vi "MongoDB.Database.CreateCollection.vi"(8 "error in (no error)":errorcluster, 11 "MongoDB.Database in":refnum<class "MongoDB.Database.lvclass">) -> (0 "error out":errorcluster, 3 "MongoDB.Database out":refnum<class "MongoDB.Database.lvclass">)   [LabVIEW 2014, in "MongoDB.Database.lvclass"]
uses:
  MongoDB.Database.lvclass
  MongoDB.Database.lvclass/MongoDB.Database.ctl
  C:/Users/Richard/Documents/GitHub/mongo-labview-driver/CSharp/bin/MongoDB.Driver.Legacy.dll
  CSharp/bin/MongoDB.Driver.Legacy.dll
panel:
  in  "collectionName":string
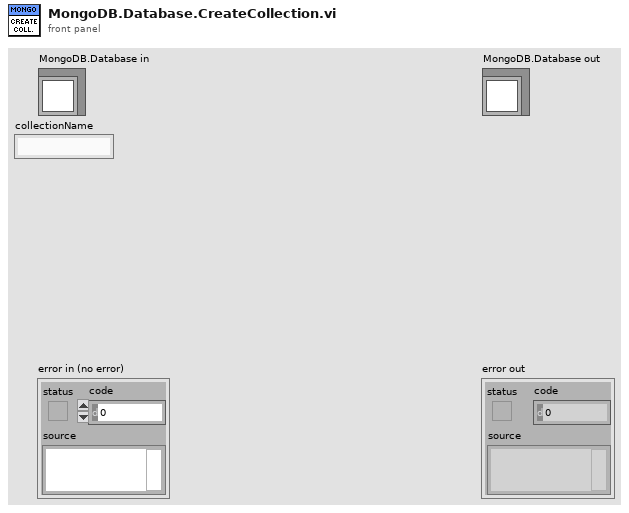
[diagram p1: front panel]
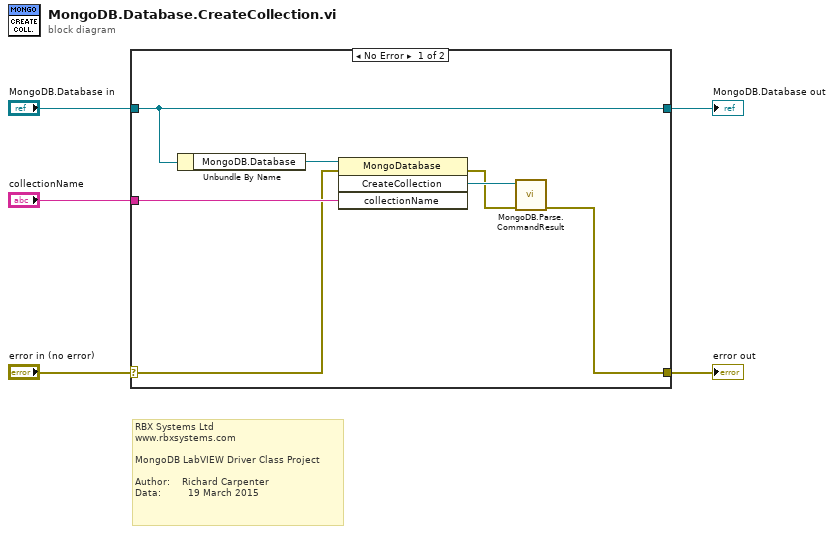
[diagram p0: block diagram]
diagram:
  # "RBX Systems Ltd\nwww.rbxsystems.com\n\nMongoDB LabVIEW Driver Class Project\n\nAuthor:    Richard Carpenter\nData:         19 March 2015"
  n1 = case shown="No Error" "error in (no error)" {
    selector: "error in (no error)" -> [w9 w14]
    tunnel: [w6 w14] -> w4
    tunnel: [w10 w13] -> w2
    tunnel: "MongoDB.Database in" -> [w10 w13]
    tunnel: "collectionName" -> [w11 _]
    frame No Error {
      n2 = Unbundle By Name(w10) -> ("MongoDB.Database"=w12:refnum<k24>)
      n3 = invoke class="MongoDatabase" method="CreateCollection"(reference=w12, error in=w9, "collectionName"=w11) -> (error out=w7:errorcluster, "CreateCollection"=w8:refnum<k24>)  [unwired: 1 in, 2 out]
      n4 = call "MongoDB.Parse.CommandResult.vi"("error in (no error)"=w7, "MongoDB.Command.Result"=w8) -> ("error out"=w6:errorcluster)  [unwired: 9 in]
    }
    frame Error {
    }
  }
  "error out" <- w4
  "MongoDB.Database out" <- w2
